vi "Writing Input Configuration File.vi"() -> ()   [LabVIEW 2022 SP3]
uses:
  source/shared/controls/digital serial audio/digital serial input settings.ctl
  <vilib>/PDM Acquisition Toolkit/shared/controls/PCM Data Justification.ctl
  <vilib>/PDM Acquisition Toolkit/shared/controls/PCM Bit Endianness.ctl
  <vilib>/PDM Acquisition Toolkit/shared/controls/Digital Edge.ctl
  source/shared/controls/master clock source.ctl
  <vilib>/PDM Acquisition Toolkit/host/Classes/Session/Controls/Logic Levels.ctl
  source/shared/controls/input type.ctl
  source/shared/controls/PDM/PDM input settings.ctl
  <vilib>/PDM Acquisition Toolkit/shared/controls/decimation order.ctl
  source/shared/controls/bit clock direction.ctl
  source/shared/input configuration file/input cfg file.lvlib
  source/shared/input configuration file/digital serial/digital serial input cfg file.lvlib
  source/shared/input configuration file/PDM/PDM input cfg file.lvlib
  <vilib>/PDM Acquisition Toolkit/shared/PDM Shared.lvlib
  <vilib>/PDM Acquisition Toolkit/host/Classes/Session/DecoderSession.lvclass
panel:
  out "input settings 2":T1={"PDM clock rate"=3072000.0, "decimation factor"=64, "bit clock direction"=enum."In", "logic level"=enum."3.3 V"} {"decimation factor" items=["24"=24, "32"=32, "48"=48, "64"=64, "96"=96, "128"=128]; "PDM clock rate" format="%#_6p"}
  in  "PDM input settings":T1={"PDM clock rate"=51200.0, "decimation factor"=1, "bit clock direction"=enum."In", "logic level"=enum."3.3 V"} {"decimation factor" items=["24"=24, "32"=32, "48"=48, "64"=64, "96"=96, "128"=128]; "PDM clock rate" format="%#_6p"}
  in  "input type 2":T5 caption="master clock source"
  out "input settings":T6={"number of channels"=51200, "data justification"=enum."Right Justified", "endianness"=enum."MSB First", "channel length"=0, "bit depth"=0, "frame clock rate"=0.0, "bit clock edge sync"=enum."Falling", "master clock source"=enum."Internal", "master clock rate"=0.0, "Logic Level"=enum."1.2 V", "frame sync edge for channel 0"=enum."Rising", "Channel 0 Offset"=0}
  out "input cfg JSON":string
  out "input type":T5 caption="master clock source"
  out "error out":errorcluster
  in  "digital serial input settings":T6={"number of channels"=0, "data justification"=enum."Left Justified", "endianness"=enum."LSB First", "channel length"=0, "bit depth"=0, "frame clock rate"=0.0, "bit clock edge sync"=enum."Falling", "master clock source"=enum."Internal", "master clock rate"=0.0, "Logic Level"=enum."1.2 V", "frame sync edge for channel 0"=enum."Rising", "Channel 0 Offset"=0}
  in  "Path":path
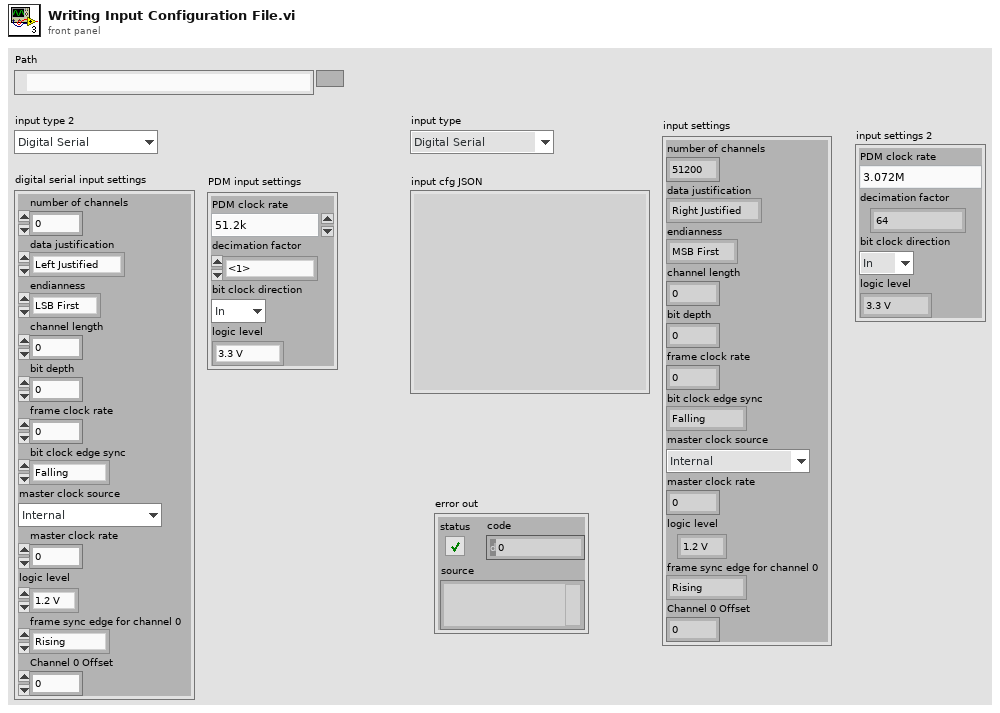
[diagram p1: front panel]
types:
  T1 = typedef "PDM input settings.ctl" = cluster{"PDM clock rate":dbl, "decimation factor":T2, "bit clock direction":T3, "logic level":T4}
  T2 = typedef "PDM Shared.lvlib/decimation order.ctl" = u16
  T3 = typedef "bit clock direction.ctl" = enum32{"In", "Out"}
  T4 = typedef "PDM Acquisition Class Library.lvlib/DecoderSession.lvclass/Logic Levels.ctl" = enum16{"3.3 V", "1.8 V", "1.2 V"}
  T5 = typedef "input type.ctl" = enum32{"Digital Serial", "PDM"}
  T6 = typedef "digital serial input settings.ctl" = cluster{"number of channels":u32, "data justification":T7, "endianness":T8, "channel length":u32, "bit depth":u32, "frame clock rate":dbl, "bit clock edge sync":T9, "master clock source":T10, "master clock rate":dbl, "Logic Level":T4, "frame sync edge for channel 0":T9, "Channel 0 Offset":u32}
  T7 = typedef "PDM Shared.lvlib/PCM Data Justification.ctl" = enum16{"Left Justified", "Right Justified"}
  T8 = typedef "PDM Shared.lvlib/PCM Bit Endianness.ctl" = enum16{"MSB First", "LSB First"}
  T9 = typedef "PDM Shared.lvlib/Digital Edge.ctl" = enum8{"Rising", "Falling"}
  T10 = typedef "master clock source.ctl" = enum32{"Internal", "External"}
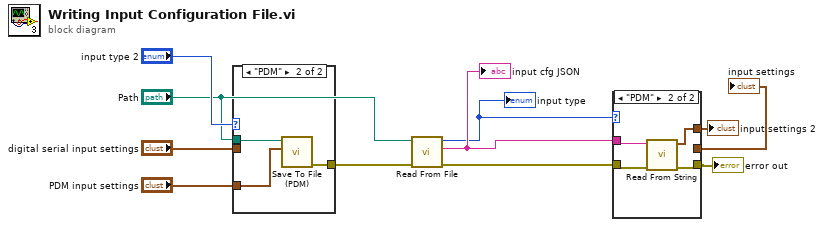
[diagram p0: block diagram]
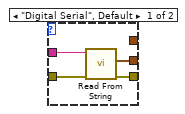
[diagram p2: hidden frame]
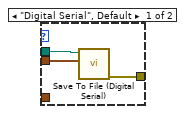
[diagram p3: hidden frame]
diagram:
  n1 = case shown="\"PDM\"" "input type 2" {
    tunnel: "digital serial input settings" -> [w14 _]
    tunnel: [w13 w17] -> w10
    tunnel: "Path" -> [w12 w16]
    tunnel: "PDM input settings" -> [_ w15]
    frame "Digital Serial", Default {
      n2 = call "Save To File (Digital Serial).vi"("digital serial input settings"=w14, "file path"=w12) -> ("error out"=w13:errorcluster)  [unwired: 9 in]
    }
    frame "PDM" {
      n3 = call "Save To File (PDM).vi"("PDM input settings"=w15, "file path"=w16) -> ("error out"=w17:errorcluster)  [unwired: 9 in]
    }
  }
  n4 = call "Read From File.vi"("error in (no error)"=w10, "file path"="Path") -> ("error out"=w9:errorcluster, "input cfg JSON"=w8:string, "input type"=w2:T5)  [unwired: 6 in, 1 out]
  "input type" <- w2
  "input cfg JSON" <- w8
  n5 = case shown="\"PDM\"" w2 {
    tunnel: w9 -> [w21 w25]
    tunnel: w8 -> [w20 w24]
    tunnel: [w19 _] -> w7
    tunnel: [w18 w23] -> w6
    tunnel: [_ w22] -> w1
    frame "Digital Serial", Default {
      n6 = call "Read From String.vi"("error in (no error)"=w21, "JSON string"=w20) -> ("error out"=w18:errorcluster, "digital serial input settings"=w19:T6)  [unwired: 8 in]
    }
    frame "PDM" {
      n7 = call "Read From String.vi"("error in (no error)"=w25, "JSON string"=w24) -> ("error out"=w23:errorcluster, "input settings"=w22:T1)  [unwired: 8 in]
    }
  }
  "error out" <- w6
  "input settings" <- w7
  "input settings 2" <- w1
